vi "Autocomplete Text.vi"(11 "Settings UI in":refnum<class "Settings UI.lvclass">) -> (3 "Settings UI out":refnum<class "Settings UI.lvclass">)   [LabVIEW 2020, in "Output Sequencer.lvlib" / "Settings UI.lvclass"]
uses:
  Settings UI.lvclass
  Settings UI.lvclass/Settings UI.ctl
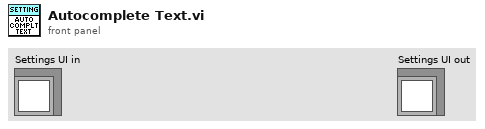
[diagram p1: front panel]
types:
  T1 = typedef "Output Sequencer.lvlib/Settings UI.lvclass/Autocomplete State.ctl" = cluster{"Variables":string[], "Active?":bool, "Search Offset":i32, "Matches":i32[], "Match Index":i32}
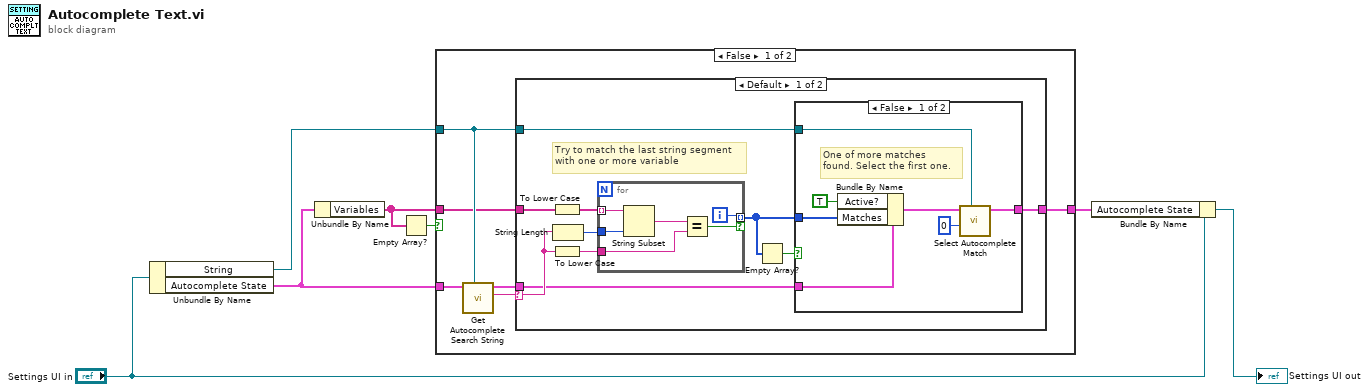
[diagram p0: block diagram]
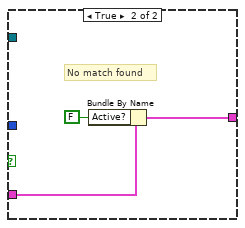
[diagram p2: hidden frame]
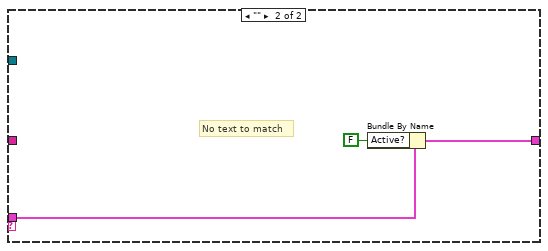
[diagram p3: hidden frame]
diagram:
  n1 = Unbundle By Name("Settings UI in") -> ("String"=w3:refnum<vi>, "Autocomplete State"=w2:T1)
  n2 = Unbundle By Name(w2) -> ("Variables"=w6:string[])
  n3 = Empty Array?(array=w6) -> (empty?=w7:bool)
  n4 = case shown="False" w7 {
    tunnel: w3 -> [w12 _]
    tunnel: [w11 w43] -> w4
    tunnel: w2 -> [w10 w43]
    tunnel: w6 -> [w8 _]
    frame False {
      n5 = call "Get Autocomplete Search String.vi"("String in"=w12, "Autocomplete State in"=w10) -> ("Search String"=w13:string, "Autocomplete State out"=w9:T1)  [unwired: 8 in]
      n6 = case shown="Default" w13 {
        selector: w13 -> [w20 _]
        tunnel: w9 -> [w18 w40]
        tunnel: w12 -> [w16 _]
        tunnel: [w15 w41] -> w11
        tunnel: w8 -> [w14 _]
        frame Default {
          # "Try to match the last string segment\nwith one or more variable"
          n7 = To Lower Case(string=w14) -> (all lower case string=w23:string[])
          n8 = To Lower Case(string=w20) -> (all lower case string=w22:string)
          n9 = String Length(string=w20) -> (length=w21:i32)
          n10 = for {
            tunnel: w22 -> [w38]
            tunnel: w23 -> [w37] mode=indexing
            tunnel: w21 -> [w36]
            tunnel: [w35] -> w19 mode=indexing if=w34
            i -> [w35]
            n11 = String Subset(string=w37, length (rest)=w36) -> (substring=w39:string)  [unwired: 1 in]
            n12 = Equal?(x=w39, y=w38) -> (x = y?=w34:bool)
          }
          n13 = Empty Array?(array=w19) -> (empty?=w17:bool)
          n14 = case shown="False" w17 {
            tunnel: w19 -> [w28 _]
            tunnel: w18 -> [w30 w33]
            tunnel: [w26 w31] -> w15
            tunnel: w16 -> [w24 _]
            frame False {
              # "One of more matches\nfound. Select the first one."
              n15 = Bundle By Name(cluster=w30, "Active?"=TRUE, "Matches"=w28) -> (w27:T1)
              n16 = call "Select Autocomplete Match.vi"("String in"=w24, "Match Index"=0, "Autocomplete State in"=w27) -> ("Autocomplete State out"=w26:T1)  [unwired: 8 in]
            }
            frame True {
              # "No match found"
              n17 = Bundle By Name(cluster=w33, "Active?"=FALSE) -> (w31:T1)
            }
          }
        }
        frame "" {
          # "No text to match"
          n18 = Bundle By Name(cluster=w40, "Active?"=FALSE) -> (w41:T1)
        }
      }
    }
    frame True {
      # "No variables to match"
    }
  }
  n19 = Bundle By Name(cluster="Settings UI in", "Autocomplete State"=w4) -> (→"Settings UI out":refnum<class "Settings UI.lvclass">)
